vi "Clear Entire Configuration - Multi FPGA.vi"(8 "error in (no error)":errorcluster, 11 "Item Ref in":T1 format="%.0x") -> (0 "error out":errorcluster)   [LabVIEW 2015, in "Engine Simulation Toolkit System Explorer.lvlib"]
uses:
  Engine Simulation Toolkit System Explorer.lvlib
  <vilib>/NI Veristand/Custom Device API/Custom Device Item Ref.ctl
  Shared/Properties.vi
  <vilib>/NI Veristand/Custom Device Tools/Custom Device Utility Library/NI VeriStand - Search for All Items by Name.vi
  <vilib>/NI Veristand/Custom Device API/Custom Device API.lvlib
  Shared/Engine Simulation Toolkit Shared.lvlib
  <vilib>/NI Veristand/Custom Device Tools/Custom Device Utility Library/Custom Device Utility Library.lvlib
panel:
  in  "RIO Name":string
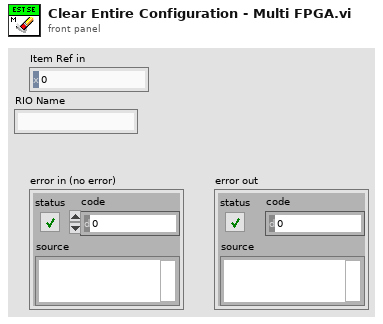
[diagram p1: front panel]
types:
  T1 = typedef "Custom Device API.lvlib/Custom Device Item Ref.ctl" = u64
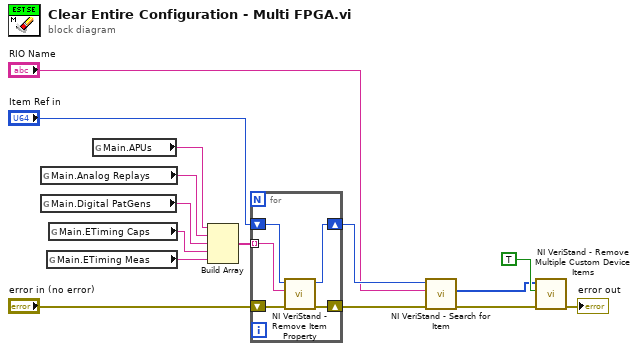
[diagram p0: block diagram]
diagram:
  n1 = global read "Properties.vi" "Main.Analog Replays"() -> (w4:string)
  n2 = global read "Properties.vi" "Main.Digital PatGens"() -> (w5:string)
  n3 = global read "Properties.vi" "Main.ETiming Meas"() -> (w7:string)
  n4 = global read "Properties.vi" "Main.ETiming Caps"() -> (w6:string)
  n5 = global read "Properties.vi" "Main.APUs"() -> (w3:string)
  n6 = Build Array(w3, w4, w5, w6, w7) -> (w2:string[])
  n7 = for {
    shift-right: [w18] -> w10
    shift-left: "error in (no error)" -> [w20]
    shift-right: [w17] -> w11
    shift-left: "Item Ref in" -> [w19]
    tunnel: w2 -> [w16] mode=indexing
    n8 = call <vilib>:"NI VeriStand - Remove Item Property.vi"("error in (no error)"=w20, "Property Name"=w16, "Item Ref in"=w19) -> ("error out"=w18:errorcluster, "Item Ref out"=w17:T1)  [unwired: 6 in, 1 out]
  }
  n9 = call-poly <vilib>:"NI VeriStand - Search for Item.vi"("error in"=w10, "Item Name"="RIO Name", "Section Ref in"=w11) -> ("error out"=w12:errorcluster, "Item Refs"=w14:T1[])  [unwired: 5 in, 2 out]
  n10 = call <vilib>:"NI VeriStand - Remove Multiple Custom Device Items.vi"("error in (no error)"=w12, "Force Delete (F)"=TRUE, "Item Refs in"=w14) -> ("error out"=→"error out":errorcluster)  [unwired: 7 in, 1 out]
